vi "Prompt for Terminal Counts.vi"(10 "Reference VI":refnum<vi>) -> (1 "Canceled?":bool, 3 "Terminal Counts":T1)   [LabVIEW 2018]
uses:
  Resource Manipulation/Terminal Counts.ctl
  Resource Manipulation.lvlib
panel:
  in  "Auto Fill":bool
  in  "Cancel":bool
  in  "OK":bool
  in  "Path":u32
  in  "String":u32
  in  "Numeric":u32
  # "How many terminals of\neach type are there, including clusters, etc.?"
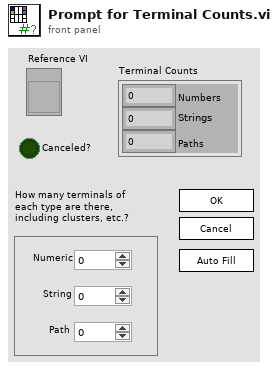
[diagram p1: front panel]
types:
  T1 = typedef "Resource Manipulation.lvlib/Terminal Counts.ctl" = cluster{"Numbers":u32, "Strings":u32, "Paths":u32}
  T2 = enum8{"Enabled", "Disabled", "Disabled and Grayed Out"}
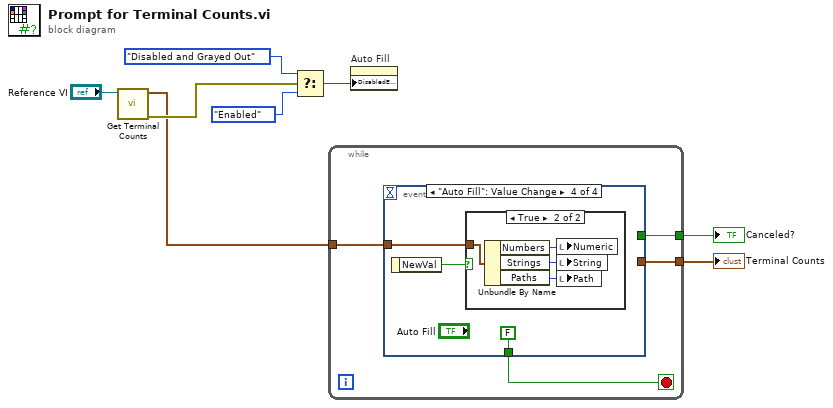
[diagram p0: block diagram]
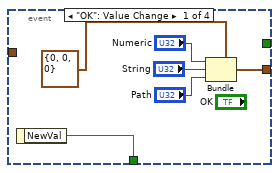
[diagram p2: hidden frame]
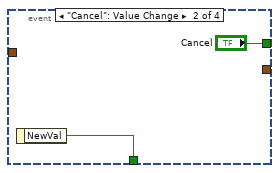
[diagram p3: hidden frame]
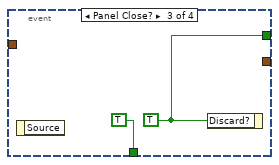
[diagram p4: hidden frame]
diagram:
  n1 = call "Get Terminal Counts.vi"("VI Refnum"="Reference VI") -> ("error out"=w2:errorcluster, "Terminal Counts"=w1:T1)  [unwired: 9 in]
  n2 = Select(t=T2."Disabled and Grayed Out" ("Disabled"), s=w2, f=T2."Enabled" ("Disabled")) -> (s? t:f=w6:T2)
  n3 = while {
    tunnel: [w12] -> w8
    tunnel: [w11] -> w7
    tunnel: w1 -> [w9]
    stop <- w10 stop-if-true
    n4 = event shown="[3] \"Auto Fill\": Value Change" {
      selector: _ -> [_ _ _ _]
      dyn-events: _ -> [_ _ _ _]
      timeout: _ -> [_ _ _ _]
      tunnel: [w15 _ _ _] -> w12
      tunnel: [_ "Cancel" w22 _] -> w11
      tunnel: [w14 w19 TRUE ("Discard?") FALSE ("Discard?")] -> w10
      tunnel: w9 -> [_ _ _ w24]
      event "OK": Value Change {
        n5 = event-data() -> ("NewVal"=w14:bool)  [unwired: 1 in]
        n6 = Bundle(cluster=T1 {"Numbers"=0, "Strings"=0, "Paths"=0} ("Terminal Counts"), "Numbers"="Numeric", "Strings"="String", "Paths"="Path") -> (w15:T1)
      }
      event "Cancel": Value Change {
        n7 = event-data() -> ("NewVal"=w19:bool)  [unwired: 1 in]
      }
      event Panel Close? {
        w22 = TRUE ("Discard?")
        n8 = event-data() -> ()  [unwired: 1 in, 1 out]
        n9 = event-data("Discard?"=w22) -> ()  [unwired: 1 in, 1 out]
      }
      event "Auto Fill": Value Change {
        n10 = event-data() -> ("NewVal"=w25:bool)  [unwired: 1 in]
        n11 = case shown="True" w25 {
          tunnel: w24 -> [_ w29]
          frame False {
          }
          frame True {
            n12 = Unbundle By Name(w29) -> ("Numbers"=w28:u32, "Strings"=w27:u32, "Paths"=w26:u32)
            n13 = local write "Numeric"(w28) -> ()
            n14 = local write "String"(w27) -> ()
            n15 = local write "Path"(w26) -> ()
          }
        }
      }
    }
  }
  "Terminal Counts" <- w8
  "Canceled?" <- w7
  n16 = property on="Auto Fill" class="Bool"("DisabledEnum"=w6) -> ()  [unwired: 2 in, 2 out]
